vi "N330X_Measure_Current.vi"(8 "error in (no error)":errorcluster, 11 "VISA Refnum in":refnum<visa-resource-name>) -> (0 "error out":errorcluster, 1 "Minimum Current":dbl, 2 "Total RMS Current":dbl, 3 "VISA Refnum out":refnum<visa-resource-name>, 4 "Maximum Current":dbl, 5 "Input Current":dbl)   [LabVIEW 2015]
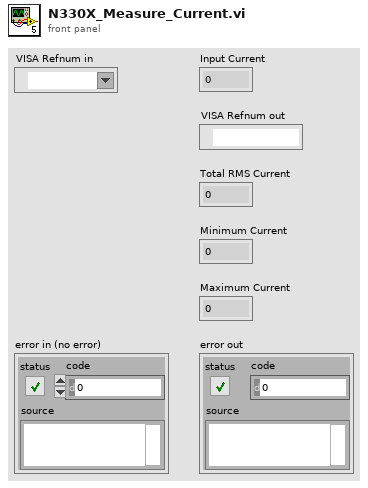
[diagram p1: front panel]
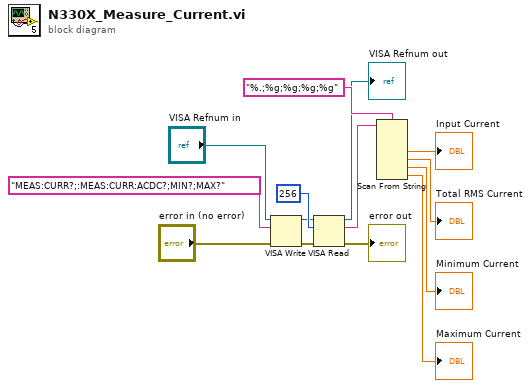
[diagram p0: block diagram]
diagram:
  n1 = VISA Write(VISA resource name="VISA Refnum in", write buffer="MEAS:CURR?;:MEAS:CURR:ACDC?;MIN?;MAX?", error in (no error)="error in (no error)") -> (VISA resource name out=w1:refnum<visa-resource-name>, error out=w3:errorcluster)  [unwired: 1 out]
  n2 = VISA Read(VISA resource name=w1, byte count=u32 256, error in (no error)=w3) -> (VISA resource name out=→"VISA Refnum out":refnum<visa-resource-name>, read buffer=w6:string, error out=→"error out":errorcluster)  [unwired: 1 out]
  n3 = Scan From String(format string="%.;%g;%g;%g;%g", input string=w6) -> (output 1=→"Input Current":dbl, output 2=→"Total RMS Current":dbl, output 3=→"Minimum Current":dbl, output 4=→"Maximum Current":dbl)  [unwired: 6 in, 3 out]
